vi "ADC INL_sweep.vi"(8 "error in (no error)":errorcluster, 9 "Sequence parameters":string[][](array[string])=[["Min limit", "Max limit", "Register sheet file", "Register Sheet"], ["", "", "CC2600.xls", "TX_BLE;Trim"], ["Reg write (addr;value)", "Operating frequency [Hz]", "", ""], ["NA", "2.44G", "", ""]], 10 "Run type":i32, 11 "Method parameters":T3={"Dev"={"Do not disturb DUT"=FALSE, "XOSC"=32000000.0, "Board type"="", "EM"="", "Configure tempboard"=TRUE, "Device specific info"=[], "Generic Object"=refnum}, "Method"={"Run type"=1, "Test name"="Current LPM2 4", "Comment"="", "Results folder"="", "AFC"=enum."Off", "Method name"="Current LPM2 4", "Method results"={"Excel brief report"=FALSE, "Spotfire report"=FALSE, "Starfish report"=FALSE}, "Operator"="", "Reference time"=timestamp(0 s since 1904-01-01), "AFC delay"=0.0, "Initialization"=enum."Enabled", "MD5 Sum"="", "HW addon board"=enum."None", "AFC Regsheet"="", "AFC Regfile"=path "", "dummy"=0.0}, "Inst"={"Instr"={"PS1"={"Name"="", "GPIB address"="", "VISA session"=""}, "PS2"={"Name"="", "GPIB address"="", "VISA session"=""}, "TC1"={"Name"="", "GPIB address"="", "VISA session"=""}, "TC2"={"Name"="", "GPIB address"="", "VISA session"=""}, "SA1"={"Name"="", "GPIB address"="", "VISA session"=""}, "SA2"={"Name"="", "GPIB address"="", "VISA session"=""}, "SG1"={"Name"="", "GPIB address"="", "VISA session"=""}, "SG2"={"Name"="", "GPIB address"="", "VISA session"=""}, "SG3"={"Name"="", "GPIB address"="", "VISA session"=""}, "MI1"={"Name"="", "GPIB address"="", "VISA session"=""}, "MI2"={"Name"="", "GPIB address"="", "VISA session"=""}, "SW SA"={"Name"="", "Controller addr"=""}, "SW SG"={"Name"="", "Controller addr"=""}, "MI3"={"Name"="", "GPIB address"="", "VISA session"=""}}, "Switchbox"={"RF Path"=0, "Cal compensation"=enum."TX", "Switchbox gain mode"="", "State"=enum."TX"}, "Instr to control (i.e. SA1)"="Default", "Intrument info string"=""}, "Sequence parameters"=[["Weight", "Min Limit", "Max Limit", "Register Sheet", "", "", "", "", "", "", "", "", ""], ["Vital", "", "1", "LPM2", "", "", "", "", "", "", "", "", ""], ["Resolution", "Reg write (addr;value)", "Chip mode", "Range", "", "", "", "", "", "", "", "", ""], ["u", "NA", "", "auto", "", "", "", "", "", "", "", "", ""]], "Cond"={"Temp logged"=25.0, "VDD1_PS1_6V"=-999.0, "VDD2_PS1_25V"=-999.0, "VDD4_PS2_25V"=-999.0, "VDD3_PS2_6V"=-999.0}, "Meas config"={"X-axis inner loop index"=32000000, "Y-axis outer loop index"=32000000, "X-axis"=[], "Y-axis"=[], "X-axis array req size"=32000000, "Y-axis array req size"=32000000, "Param description"=[], "Use meas clust for reporting"=FALSE, "Parameter index (page)"=0, "X-axis name"="", "Y-axis name"=""}} {"Cond"."VDD3_PS2_6V" format="%.3f"; "Cond"."VDD4_PS2_25V" format="%.3f"; "Cond"."VDD2_PS1_25V" format="%.3f"; "Cond"."VDD1_PS1_6V" format="%.3f"; "Method"."dummy" format="%.1p"; "Method"."AFC delay" format="%.1p"; "Dev"."XOSC" format="%.3p"}) -> (0 "error out":errorcluster, 1 "End method error":T2, 2 "Short Results":string[](array[string])=["0.00", "0.00", "0.00", "0.00"], 3 "Result summary":string[][](array[string])=[["Critical", "Output Power@2405 MHz", "-3", "4", "dBm"], ["Critical", "Output Power@2410 MHz", "-3", "4", "dBm"]])   [LabVIEW 2019]
doc: "[AutoDocStart]Performs crystal accuracy measurements. Measures the offset from ideal frequency. Primarily used for tuning XOSC capacitors and verifying XOSC trims.\n\nSweeping parameters: operating frequency, OSC override value and VDDR level\n\nResults: Offset frequency in ppm[AutoDocEnd]"
uses:
  User Lib/Utilities/Cluster definitions/DUT VDD1.ctl
  User Lib/Utilities/Cluster definitions/DUT VDD2.ctl
  User Lib/Utilities/Cluster definitions/DUT VDD3.ctl
  User Lib/Utilities/Cluster definitions/DUT VDD4.ctl
  User Lib/Utilities/Cluster definitions/DUT vdd control.ctl
  42f514b6-df04-40b6-a03b-a487344522a2.vi
  3f8b4189-43b3-45b7-8bba-bb7e10ae7045.vi
  47332434-656c-4693-9234-e05a15154894.vi
  62b45376-0a3e-4237-a030-b0a612edc8e5.vi
  b7ff9f93-cf4b-49d2-9220-d5c2ebaf56eb.vi
  9f9df643-cad2-47cb-a2d6-a9993951f146.vi
  0285ada5-cea9-4f7c-8e18-3c0901f4aec6.vi
  d5327cad-c336-4ca6-ac46-e2641e1e3ffd.vi
  User Lib/Utilities/Cluster definitions/Instr clust.ctl
  User Lib/Utilities/Cluster definitions/Method input.ctl
  User Lib/Utilities/Controls/Automatic Frequency Compensation types.ctl
  User Lib/Utilities/Controls/Method Reports.ctl
  User Lib/Utilities/Cluster definitions/End method error cluster.ctl
  User Lib/Utilities/Cluster definitions/Device specific info.ctl
  User Lib/Utilities/Cluster definitions/Method Initialization.ctl
  User Lib/Utilities/Switchbox control/SwitchBox_State._ENUMctl.ctl
  User Lib/Utilities/Controls/HW addon boards.ctl
panel:
  in  "Tab Control":T1(tab)
  # "°C"
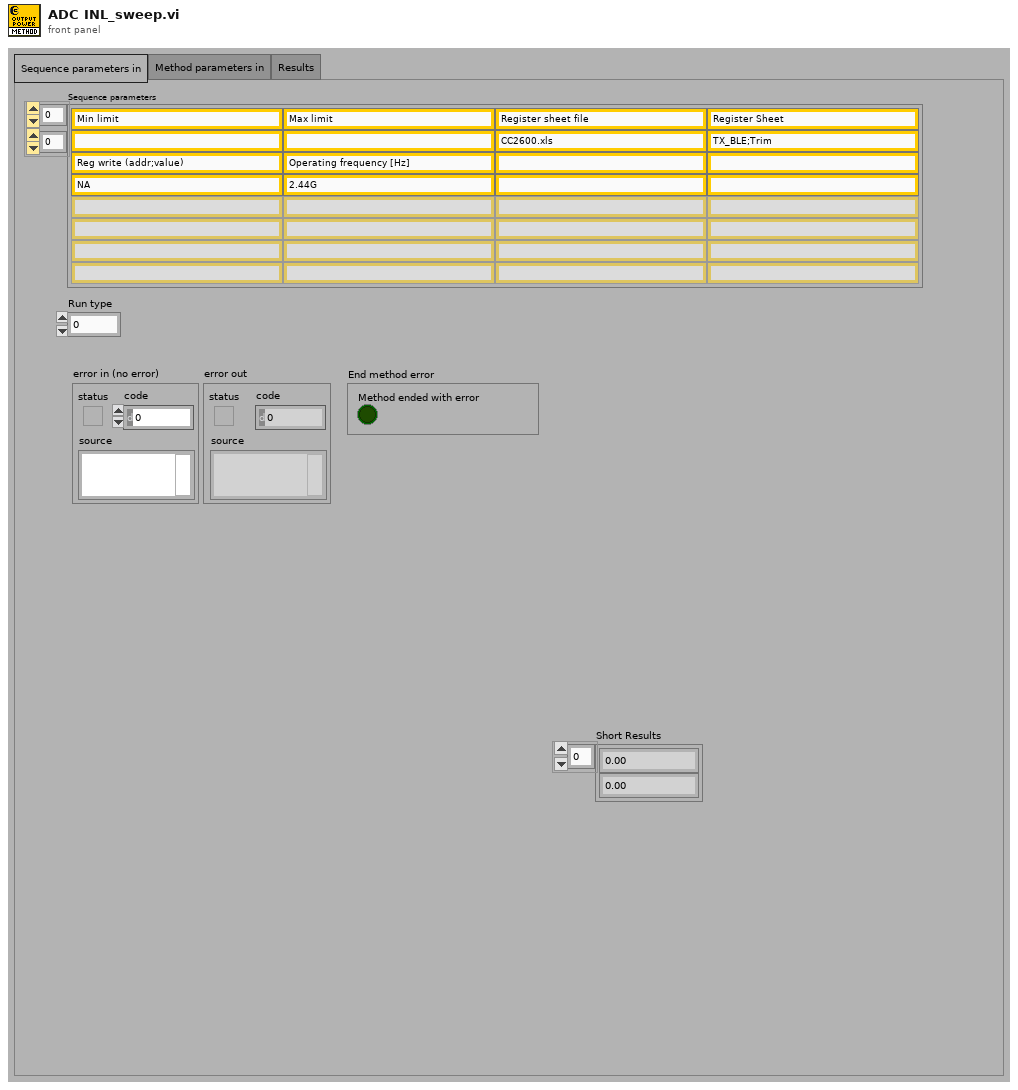
[diagram p1: front panel]
types:
  T1 = enum32{"Sequence parameters in", "Method parameters in", "Results"}
  T2 = typedef "End method error cluster.ctl" = cluster{"Method ended with error":bool}
  T3 = typedef "Method input.ctl" = cluster{"Dev":cluster{"Do not disturb DUT":bool, "XOSC":dbl, "Board type":string, "EM":string, "Configure tempboard":bool, "Device specific info":T4[], "Generic Object":refnum<class>}, "Method":cluster{"Run type":i32, "Test name":string, "Comment":string, "Results folder":string, "AFC":T5, "Method name":string, "Method results":T6, "Operator":string, "Reference time":timestamp, "AFC delay":dbl, "Initialization":T7, "MD5 Sum":string, "HW addon board":T8, "AFC Regsheet":string, "AFC Regfile":path, "dummy":dbl}, "Inst":T9, "Sequence parameters":string[][], "Cond":cluster{"Temp logged":dbl, "VDD1_PS1_6V":dbl, "VDD2_PS1_25V":dbl, "VDD4_PS2_25V":dbl, "VDD3_PS2_6V":dbl}, "Meas config":cluster{"X-axis inner loop index":i32, "Y-axis outer loop index":i32, "X-axis":string[], "Y-axis":string[], "X-axis array req size":i32, "Y-axis array req size":i32, "Param description":string[][], "Use meas clust for reporting":bool, "Parameter index (page)":i32, "X-axis name":string, "Y-axis name":string}}
  T4 = typedef "Device specific info.ctl" = cluster{"EM number":u8, "IP address":string, "Enabled":bool, "Slot no":u8, "RF path":u8, "EM name":string, "Wafer info":string, "AFC frequency ppm":dbl, "Register writes":string[][], "Meas data":string[][][], "Device comment":string}
  T5 = typedef "Automatic Frequency Compensation types.ctl" = enum16{"Off", "Compensate Instrument frequency", "Compensate DUT frequency", "Predictive - Compensate Instrument frequency", "Predictive - Compensate DUT frequency", "Do not skip re-init - Compensate Instrument frequency", "Do not skip re-init - Compensate DUT frequency"}
  T6 = typedef "Method Reports.ctl" = cluster{"Excel brief report":bool, "Spotfire report":bool, "Starfish report":bool}
  T7 = typedef "Method Initialization.ctl" = enum16{"Enabled", "Skip Instr and Device Init", "Enabled with Separate Flash", "Set PS, Device Init and Skip Instr Init", "Skip Device Init"}
  T8 = typedef "HW addon boards.ctl" = enum16{"None", "Current meas 5EM", "Stresstest 10EM"}
  T9 = typedef "Instr clust.ctl" = cluster{"Instr":cluster{"PS1":cluster{"Name":string, "GPIB address":string, "VISA session":refnum<visa-resource-name>}, "PS2":cluster{"Name":string, "GPIB address":string, "VISA session":refnum<visa-resource-name>}, "TC1":cluster{"Name":string, "GPIB address":string, "VISA session":refnum<visa-resource-name>}, "TC2":cluster{"Name":string, "GPIB address":string, "VISA session":refnum<visa-resource-name>}, "SA1":cluster{"Name":string, "GPIB address":string, "VISA session":refnum<visa-resource-name>}, "SA2":cluster{"Name":string, "GPIB address":string, "VISA session":refnum<visa-resource-name>}, "SG1":cluster{"Name":string, "GPIB address":string, "VISA session":refnum<visa-resource-name>}, "SG2":cluster{"Name":string, "GPIB address":string, "VISA session":refnum<visa-resource-name>}, "SG3":cluster{"Name":string, "GPIB address":string, "VISA session":refnum<visa-resource-name>}, "MI1":cluster{"Name":string, "GPIB address":string, "VISA session":refnum<visa-resource-name>}, "MI2":cluster{"Name":string, "GPIB address":string, "VISA session":refnum<visa-resource-name>}, "SW SA":cluster{"Name":string, "Controller addr":string}, "SW SG":cluster{"Name":string, "Controller addr":string}, "MI3":cluster{"Name":string, "GPIB address":string, "VISA session":refnum<visa-resource-name>}}, "Switchbox":cluster{"RF Path":i32, "Cal compensation":enum16{"TX", "RX", "Interferer", "No compensation", "Interferer2"}, "Switchbox gain mode":string, "State":T10}, "Instr to control (i.e. SA1)":string, "Intrument info string":string}
  T10 = typedef "SwitchBox_State._ENUMctl.ctl" = enum16{"TX", "RX", "SP:TX", "SP:RX", "SW:TX", "SW:RX"}
  T11 = typedef "DUT vdd control.ctl" = cluster{"VDD4 config":T12, "VDD3 config":T13, "VDD2 config":T14, "VDD1 config":T15}
  T12 = typedef "DUT VDD4.ctl" = u16
  T13 = typedef "DUT VDD3.ctl" = u16
  T14 = typedef "DUT VDD2.ctl" = u16
  T15 = typedef "DUT VDD1.ctl" = u16
  T16 = enum32{"NI Card Settings", "Memory Read Setting", "DC Capture", "ADC Ramp", "ADC Sine", "SNR", "Cap Calibration"}
  T17 = enum32{"Read from Memory", "Read .dat file", "NI Card Capture", "None"}
  T18 = cluster{"Path to Save plot":path, "Path to Raw Data plot":path}
  T19 = cluster{"Save INL/DNL Plot(Ramp)":bool, "Save SNR Plot":bool, "Save INL/DNL Plot(Sine)":bool, "Save INL/DNL Raw Data(Ramp)":bool, "Save SNR Raw Data":bool, "Save INL/DNL Raw Data(Sine)":bool, "Save DC Raw data":bool, "Save  Raw Data(Sine)":bool}
  T20 = cluster{"Min INL":dbl, "Max INL":dbl, "Min DNL":dbl, "Max DNL":dbl, "INL Range":dbl, "DNL Range":dbl, "Avg Hits/Code":dbl}
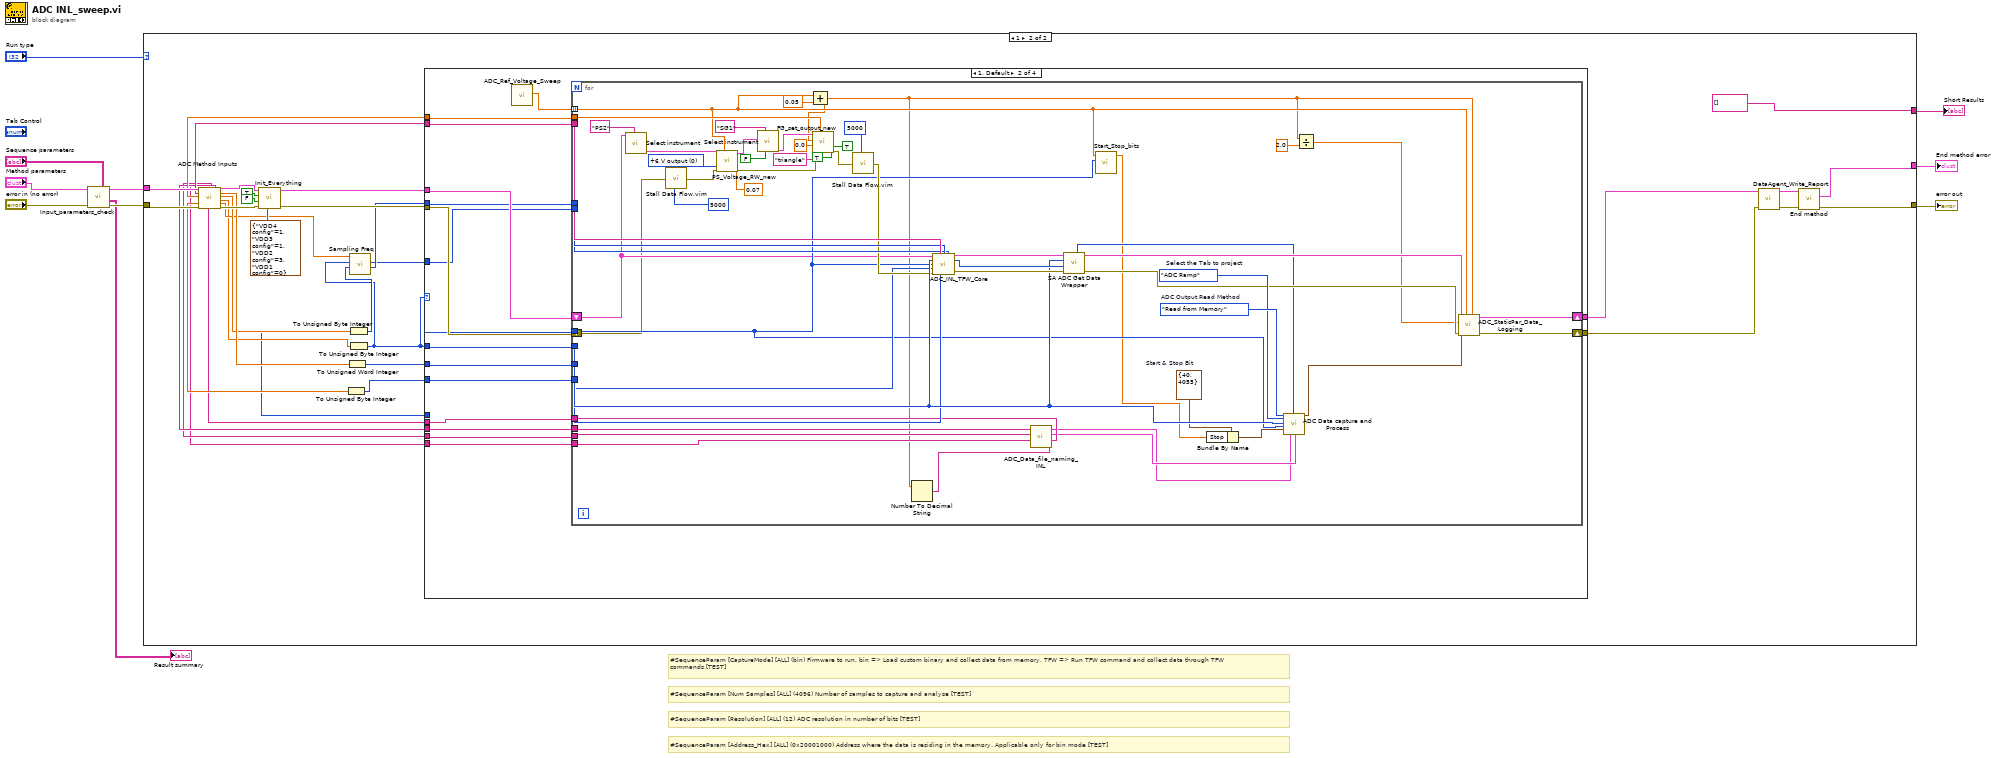
[diagram p0: block diagram]
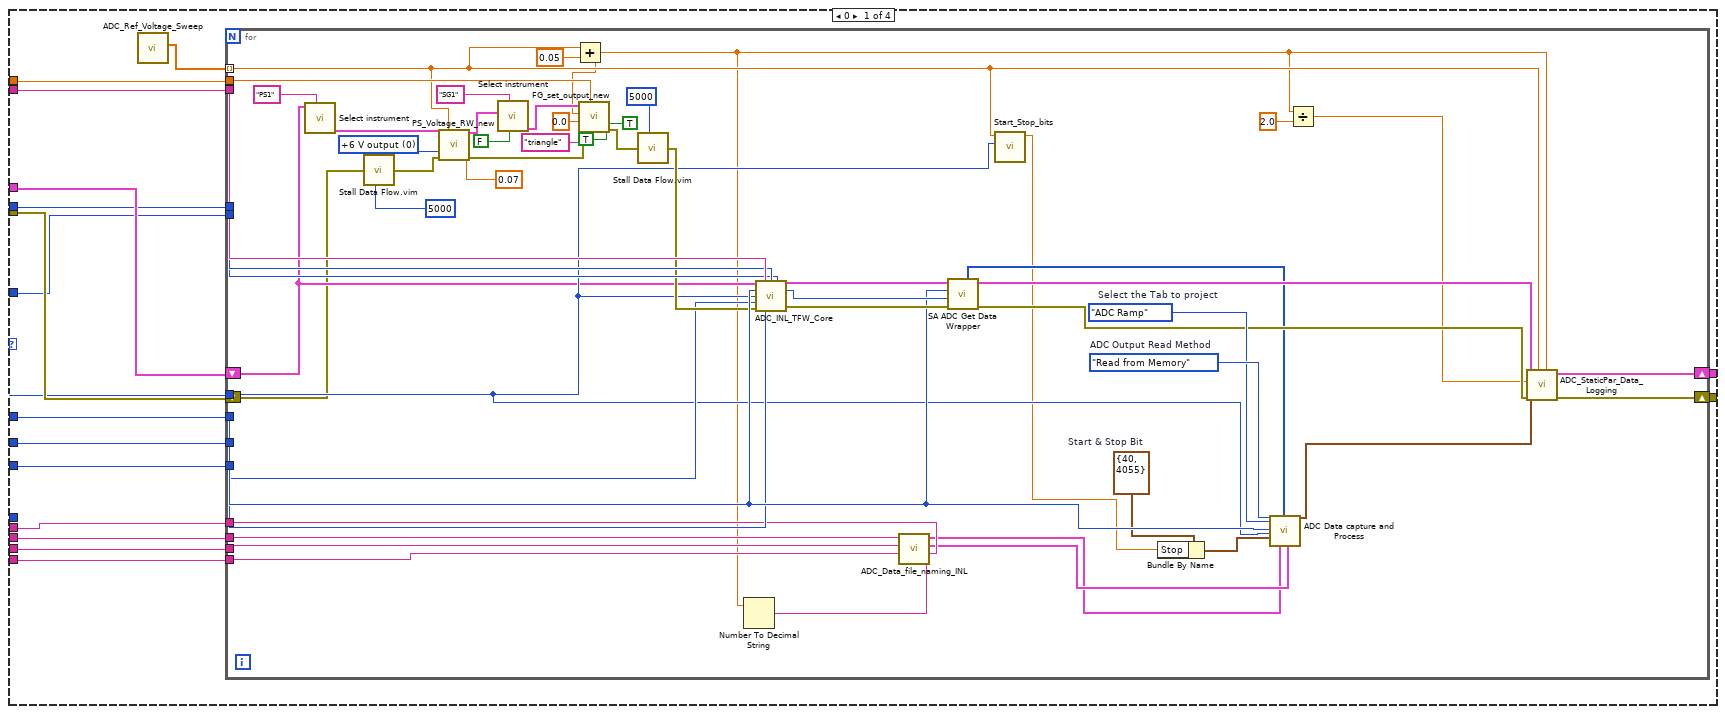
[diagram p3: hidden frame]
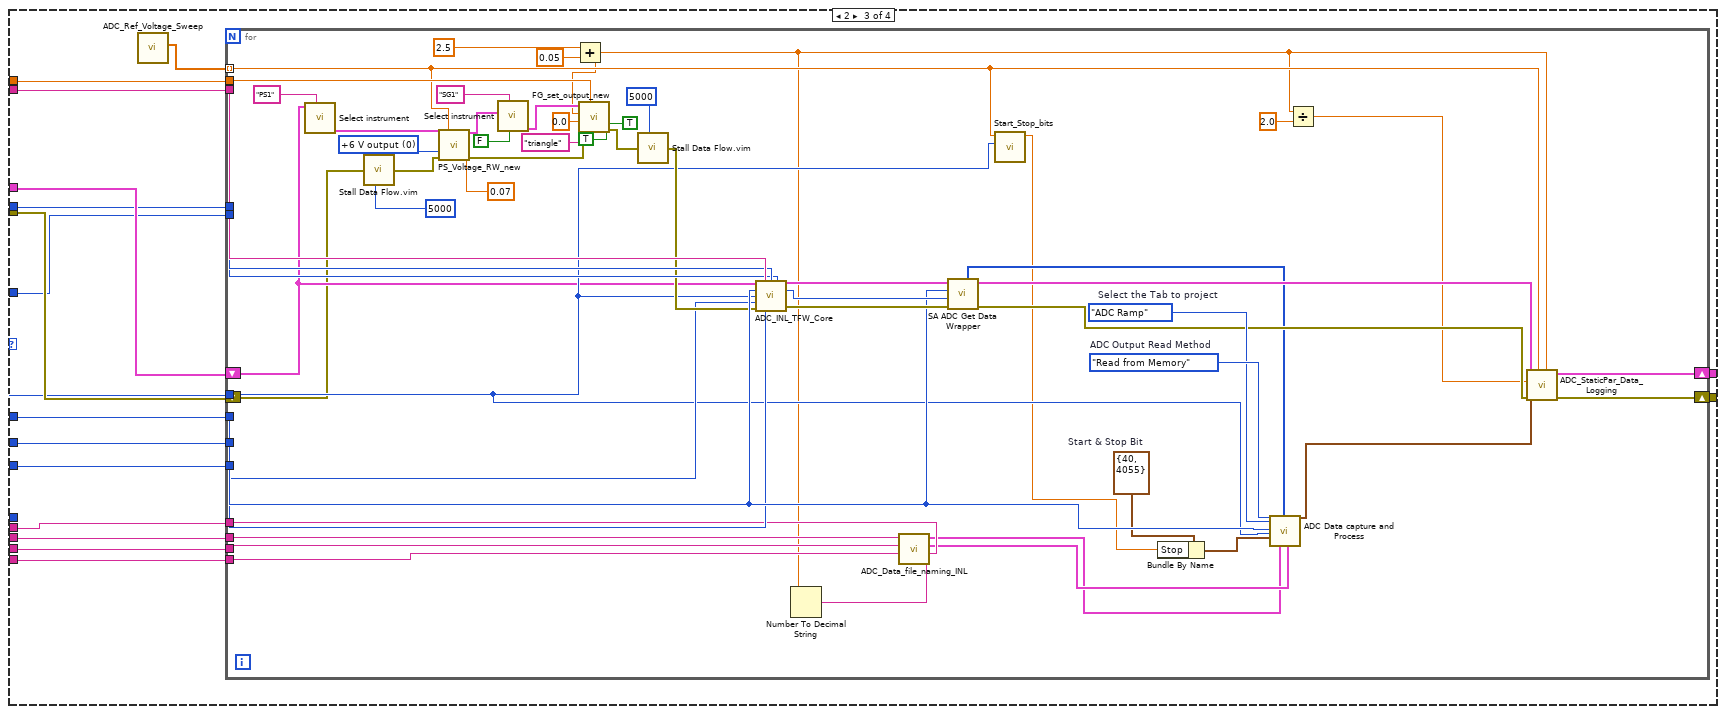
[diagram p4: hidden frame]
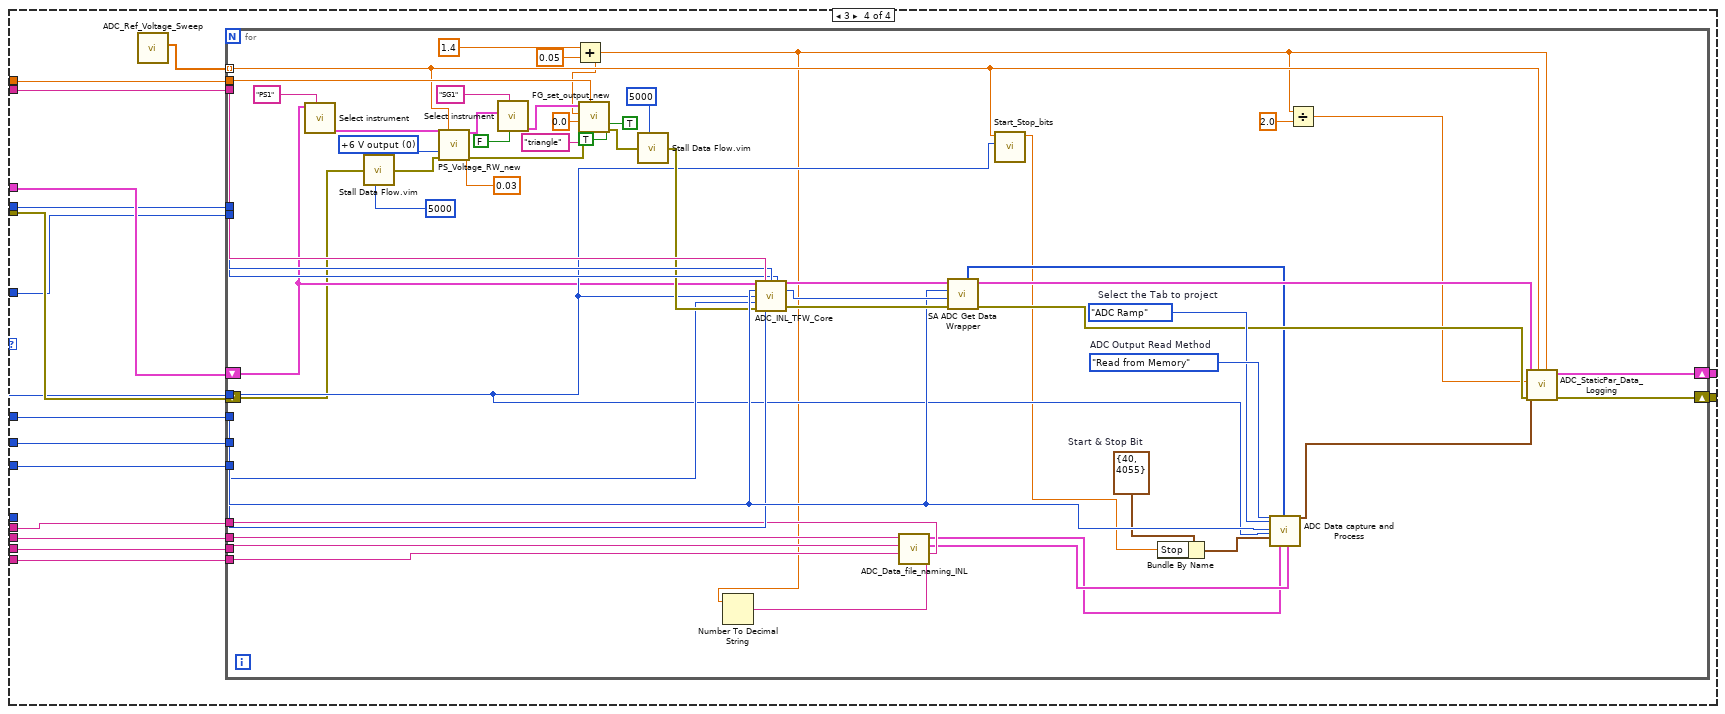
[diagram p5: hidden frame]
diagram:
  # "#SequenceParam [Num Samples] [ALL] (4096) Number of samples to capture and analyse [TEST]"
  # "#SequenceParam [CaptureMode] [ALL] (bin) Firmware to run. bin => Load custom binary and collect data from memory. TFW => Run TFW command and collect data through TFW commands [TEST]"
  # "#SequenceParam [Address_Hex] [ALL] (0x20001000) Address where the data is residing in the memory. Applicable only for bin mode [TEST]"
  # "#SequenceParam [Resolution] [ALL] (12) ADC resolution in number of bits [TEST]"
  n1 = call "Input_parameters_check.vi"("Sequence parameters"="Sequence parameters", "error in"="error in (no error)", "Method cluster in"="Method parameters") -> ("error out"=w9:errorcluster, "Result summary"=→"Result summary":string[][], "Method cluster out"=w5:T3)  [unwired: 6 in]
  n2 = case shown="1" "Run type" {
    tunnel: w9 -> [w11 w33]
    tunnel: [w11 w44] -> w10
    tunnel: w5 -> [_ w34]
    tunnel: [_ w43] -> w4
    tunnel: [_ string[] []] -> w1
    frame 0, Default {
      # "Run type 0 is only for formatting the result summary"
    }
    frame 1 {
      n3 = call "ADC Method Inputs.vi"("Method cluster in"=w34, "error in (no error)"=w33) -> ("Capture Mode"=w21:string, "Signal Freq"=w17:dbl, "ADC Chnl No."=w26:dbl, "Sampling Freq String"=w14:string, "Chnl No. string"=w13:string, "Resolution String"=w15:string, "Voltage Ref String"=w16:string, "Method cluster out"=w31:T3, "Num Samples"=w30:dbl, "Resolution"=w29:dbl, "Voltage Ref"=w27:dbl, "Sampling Freq"=w28:dbl, "error out"=w32:errorcluster)  [unwired: 3 in, 2 out]
      n4 = call "Init_Everything.vi"("VDD config"=T11 {"VDD4 config"=1, "VDD3 config"=1, "VDD2 config"=3, "VDD1 config"=0}, "error in"=w32, "Support current measurement?"=FALSE, "Override VDD Config"=TRUE, "Method cluster In"=w31) -> ("error out"=w25:errorcluster, "Method cluster out"=w12:T3)  [unwired: 3 in, 2 out]
      n5 = To Unsigned Byte Integer(number=w26) -> (unsigned 8bit integer=w22:u8)
      n6 = To Unsigned Word Integer(number=w30) -> (unsigned 16bit integer=w24:u16)
      n7 = To Unsigned Byte Integer(number=w29) -> (unsigned 8bit integer=w23:u8)
      n8 = To Unsigned Byte Integer(number=w27) -> (unsigned 8bit integer=w18:u8)
      n9 = call "Sampling Freq.vi"("Resolution"=w23, "Voltage Ref"=w18, "Sampling Freq"=w28) -> ("LGPT Count"=w20:u16, "SCOMP"=w19:u16)  [unwired: 7 in]
      n10 = case shown="1, Default" w18 {
        tunnel: [w61 w132 w203 w275] -> w38
        tunnel: [w60 w131 w202 w274] -> w37
        tunnel: w12 -> [w59 w130 w201 w273]
        tunnel: w25 -> [w58 w129 w200 w272]
        tunnel: w24 -> [w57 w128 w199 w271]
        tunnel: w23 -> [w56 w127 w198 w270]
        tunnel: w18 -> [w55 w126 w197 w269]
        tunnel: w22 -> [w54 w125 w196 w268]
        tunnel: w21 -> [w53 w124 w195 w267]
        tunnel: w20 -> [w52 w123 w194 w266]
        tunnel: w19 -> [w51 w122 w193 w265]
        tunnel: w17 -> [w49 w120 w191 w263]
        tunnel: w16 -> [w48 w119 w190 w262]
        tunnel: w15 -> [w47 w118 w189 w261]
        tunnel: w14 -> [w46 w117 w188 w260]
        tunnel: w13 -> [w45 w116 w187 w259]
        frame 0 {
          n11 = call "ADC_Ref_Voltage_Sweep.vi"() -> ("Ref voltage sweep"=w50:dbl[])  [unwired: 11 in]
          n12 = for {
            tunnel: w57 -> [w104]
            tunnel: w56 -> [w82]
            tunnel: w55 -> [w83]
            tunnel: w54 -> [w103]
            tunnel: w53 -> [w102]
            tunnel: w52 -> [w101]
            tunnel: w51 -> [w100]
            shift-right: [w110] -> w61
            shift-left: w59 -> [w76]
            shift-right: [w109] -> w60
            shift-left: w58 -> [w70]
            tunnel: w50 -> [w65] mode=indexing
            tunnel: w49 -> [w92]
            tunnel: w48 -> [w89]
            tunnel: w47 -> [w88]
            tunnel: w46 -> [w87]
            tunnel: w45 -> [w86]
            w77 = u16 0 items=["+6 V output", "+25 V output", "-25 V output", "ALL TERM"] ("Output Terminals")
            w81 = cluster{"Start":i32, "Stop":i32} {"Start"=40, "Stop"=4055}  # Start & Stop Bit
            w114 = T16."ADC Ramp"  # Select the Tab to project
            w115 = T17."Read from Memory"  # ADC Output Read Method
            n13 = call "Select instrument.vi"("Instr.Instr to control (i.e. SA1)"="PS1", "Method cluster in"=w76) -> ("Instr out"=w75:T9)  [unwired: 7 in, 2 out]
            n14 = call "Stall Data Flow.vim"("value in"=w70, "milliseconds to wait"=u32 5000) -> ("value out"=w71:errorcluster)  [unwired: 1 out]
            n15 = call "PS_Voltage_RW_new.vi"("InstrCluster in"=w75, "Set Voltage"=w65, "Current(0)"=0.07, "Output Terminals"=w77, "error in (no error)"=w71) -> ("InstrCluster out"=w74:T9, "error out"=w78:errorcluster)  [unwired: 8 in, 1 out]
            n16 = call "Select instrument.vi"("Method cluster (T) / Instr cluster (F)"=FALSE, "Instr.Instr to control (i.e. SA1)"="SG1", "Instr in"=w74) -> ("Instr out"=w99:T9)  [unwired: 6 in, 2 out]
            n17 = Add(x=w65, y=0.05) -> (x+y=w63:dbl)
            n18 = call "FG_set_output_new.vi"("High impedance (T)"=TRUE, "Enable Output?"=TRUE, "Function (DC, Sine, Square, Triangle, Ramp up, Ramp down, Pulse)"="triangle", "Frequency [Hz]"=w92, "error in"=w78, "Low voltage"=0.0, "High voltage (or DC)"=w63, "InstrCluster in"=w99) -> ("error out"=w97:errorcluster)  [unwired: 2 in, 1 out]
            n19 = call "Stall Data Flow.vim"("value in"=w97, "milliseconds to wait"=u32 5000) -> ("value out"=w96:errorcluster)  [unwired: 1 out]
            n20 = Number To Decimal String(number=w63) -> (decimal integer string=w64:string)  [unwired: 1 in]
            n21 = call "ADC_INL_TFW_Core.vi"("Method cluster in"=w76, "Capture Mode"=w102, "LGPT Count"=w101, "SCOMP"=w100, "No. Samples"=w104, "Resolution"=w82, "Voltage Ref"=w83, "error in"=w96, "ADC Chnl No."=w103) -> ("Method cluster out"=w106:T3, "ResPar[0] Data Address"=w105:u32, "error out"=w107:errorcluster)  [unwired: 3 in, 1 out]
            n22 = call "ADC_Data_file_naming_INL.vi"("Amplitude (Vpp)"=w64, "ADC Chn. No"=w86, "Sampling Freq String"=w87, "Resolution String"=w88, "Voltage Ref String"=w89) -> ("path to save"=w85:T18, "Save data"=w84:T19)  [unwired: 5 in]
            n23 = call "SA ADC Get Data Wrapper.vi"("error in"=w107, "Data Address"=w105, "Num Samples"=w104, "Method cluster in"=w106) -> ("error out"=w113:errorcluster, "output cluster"=w112:T3, "ADC samples"=w111:u32[])  [unwired: 2 in, 3 out]
            n24 = call "Start_Stop_bits.vi"("Resolution"=w82, "Input Amplitude"=w65) -> ("Stop Bit"=w79:dbl)  [unwired: 9 in]
            n25 = Bundle By Name(cluster=w81, "Stop"=w79) -> (w80:cluster{"Start":i32, "Stop":i32})
            n26 = call "ADC Data capture and Process.vi"("ADC Output Read Method"=w115, "Select the Tab to project"=w114, "No.of samples"=w104, "Resolution"=w82, "Start & Stop Bit"=w80, "Save data"=w84, "Input Waveform"=w111, "path to save"=w85) -> ("Static Parameters (Ramp)"=w108:T20)  [unwired: 14 in, 5 out]
            n27 = Divide(x=w63, y=2.0) -> (x/y=w67:dbl)
            n28 = call "ADC_StaticPar_Data_Logging.vi"("Offset (V)"=w67, "Amplitude (Vpp)"=w63, "Ref Voltage"=w65, "error in (no error)"=w113, "Static Parameters (Ramp)"=w108, "output cluster"=w112) -> ("error out"=w109:errorcluster, "Method cluster out"=w110:T3)  [unwired: 4 in]
          }
        }
        frame 1, Default {
          n29 = call "ADC_Ref_Voltage_Sweep.vi"() -> ("Ref voltage sweep"=w121:dbl[])  [unwired: 11 in]
          n30 = for {
            tunnel: w128 -> [w175]
            tunnel: w127 -> [w153]
            tunnel: w126 -> [w154]
            tunnel: w125 -> [w174]
            tunnel: w124 -> [w173]
            tunnel: w123 -> [w172]
            tunnel: w122 -> [w171]
            shift-right: [w181] -> w132
            shift-left: w130 -> [w147]
            shift-right: [w180] -> w131
            shift-left: w129 -> [w141]
            tunnel: w121 -> [w136] mode=indexing
            tunnel: w120 -> [w163]
            tunnel: w119 -> [w160]
            tunnel: w118 -> [w159]
            tunnel: w117 -> [w158]
            tunnel: w116 -> [w157]
            w148 = u16 0 items=["+6 V output", "+25 V output", "-25 V output", "ALL TERM"] ("Output Terminals")
            w152 = cluster{"Start":i32, "Stop":i32} {"Start"=40, "Stop"=4055}  # Start & Stop Bit
            w185 = T16."ADC Ramp"  # Select the Tab to project
            w186 = T17."Read from Memory"  # ADC Output Read Method
            n31 = call "Select instrument.vi"("Instr.Instr to control (i.e. SA1)"="PS2", "Method cluster in"=w147) -> ("Instr out"=w146:T9)  [unwired: 7 in, 2 out]
            n32 = call "Stall Data Flow.vim"("value in"=w141, "milliseconds to wait"=u32 5000) -> ("value out"=w142:errorcluster)  [unwired: 1 out]
            n33 = call "PS_Voltage_RW_new.vi"("InstrCluster in"=w146, "Set Voltage"=w136, "Current(0)"=0.07, "Output Terminals"=w148, "error in (no error)"=w142) -> ("InstrCluster out"=w145:T9, "error out"=w149:errorcluster)  [unwired: 8 in, 1 out]
            n34 = call "Select instrument.vi"("Method cluster (T) / Instr cluster (F)"=FALSE, "Instr.Instr to control (i.e. SA1)"="SG1", "Instr in"=w145) -> ("Instr out"=w170:T9)  [unwired: 6 in, 2 out]
            n35 = Add(x=w136, y=0.05) -> (x+y=w134:dbl)
            n36 = call "FG_set_output_new.vi"("High impedance (T)"=TRUE, "Enable Output?"=TRUE, "Function (DC, Sine, Square, Triangle, Ramp up, Ramp down, Pulse)"="triangle", "Frequency [Hz]"=w163, "error in"=w149, "Low voltage"=0.0, "High voltage (or DC)"=w134, "InstrCluster in"=w170) -> ("error out"=w168:errorcluster)  [unwired: 2 in, 1 out]
            n37 = call "Stall Data Flow.vim"("value in"=w168, "milliseconds to wait"=u32 5000) -> ("value out"=w167:errorcluster)  [unwired: 1 out]
            n38 = Number To Decimal String(number=w134) -> (decimal integer string=w135:string)  [unwired: 1 in]
            n39 = call "ADC_INL_TFW_Core.vi"("Method cluster in"=w147, "Capture Mode"=w173, "LGPT Count"=w172, "SCOMP"=w171, "No. Samples"=w175, "Resolution"=w153, "Voltage Ref"=w154, "error in"=w167, "ADC Chnl No."=w174) -> ("Method cluster out"=w177:T3, "ResPar[0] Data Address"=w176:u32, "error out"=w178:errorcluster)  [unwired: 3 in, 1 out]
            n40 = call "ADC_Data_file_naming_INL.vi"("Amplitude (Vpp)"=w135, "ADC Chn. No"=w157, "Sampling Freq String"=w158, "Resolution String"=w159, "Voltage Ref String"=w160) -> ("path to save"=w156:T18, "Save data"=w155:T19)  [unwired: 5 in]
            n41 = call "SA ADC Get Data Wrapper.vi"("error in"=w178, "Data Address"=w176, "Num Samples"=w175, "Method cluster in"=w177) -> ("error out"=w184:errorcluster, "output cluster"=w183:T3, "ADC samples"=w182:u32[])  [unwired: 2 in, 3 out]
            n42 = call "Start_Stop_bits.vi"("Resolution"=w153, "Input Amplitude"=w136) -> ("Stop Bit"=w150:dbl)  [unwired: 9 in]
            n43 = Bundle By Name(cluster=w152, "Stop"=w150) -> (w151:cluster{"Start":i32, "Stop":i32})
            n44 = call "ADC Data capture and Process.vi"("ADC Output Read Method"=w186, "Select the Tab to project"=w185, "No.of samples"=w175, "Resolution"=w153, "Start & Stop Bit"=w151, "Save data"=w155, "Input Waveform"=w182, "path to save"=w156) -> ("Static Parameters (Ramp)"=w179:T20)  [unwired: 14 in, 5 out]
            n45 = Divide(x=w134, y=2.0) -> (x/y=w138:dbl)
            n46 = call "ADC_StaticPar_Data_Logging.vi"("Offset (V)"=w138, "Amplitude (Vpp)"=w134, "Ref Voltage"=w136, "error in (no error)"=w184, "Static Parameters (Ramp)"=w179, "output cluster"=w183) -> ("error out"=w180:errorcluster, "Method cluster out"=w181:T3)  [unwired: 4 in]
          }
        }
        frame 2 {
          n47 = call "ADC_Ref_Voltage_Sweep.vi"() -> ("Ref voltage sweep"=w192:dbl[])  [unwired: 11 in]
          n48 = for {
            tunnel: w199 -> [w247]
            tunnel: w198 -> [w225]
            tunnel: w197 -> [w226]
            tunnel: w196 -> [w246]
            tunnel: w195 -> [w245]
            tunnel: w194 -> [w244]
            tunnel: w193 -> [w243]
            shift-right: [w253] -> w203
            shift-left: w201 -> [w219]
            shift-right: [w252] -> w202
            shift-left: w200 -> [w213]
            tunnel: w192 -> [w208] mode=indexing
            tunnel: w191 -> [w235]
            tunnel: w190 -> [w232]
            tunnel: w189 -> [w231]
            tunnel: w188 -> [w230]
            tunnel: w187 -> [w229]
            w220 = u16 0 items=["+6 V output", "+25 V output", "-25 V output", "ALL TERM"] ("Output Terminals")
            w224 = cluster{"Start":i32, "Stop":i32} {"Start"=40, "Stop"=4055}  # Start & Stop Bit
            w257 = T16."ADC Ramp"  # Select the Tab to project
            w258 = T17."Read from Memory"  # ADC Output Read Method
            n49 = call "Select instrument.vi"("Instr.Instr to control (i.e. SA1)"="PS1", "Method cluster in"=w219) -> ("Instr out"=w218:T9)  [unwired: 7 in, 2 out]
            n50 = call "Stall Data Flow.vim"("value in"=w213, "milliseconds to wait"=u32 5000) -> ("value out"=w214:errorcluster)  [unwired: 1 out]
            n51 = call "PS_Voltage_RW_new.vi"("InstrCluster in"=w218, "Set Voltage"=w208, "Current(0)"=0.07, "Output Terminals"=w220, "error in (no error)"=w214) -> ("InstrCluster out"=w217:T9, "error out"=w221:errorcluster)  [unwired: 8 in, 1 out]
            n52 = call "Select instrument.vi"("Method cluster (T) / Instr cluster (F)"=FALSE, "Instr.Instr to control (i.e. SA1)"="SG1", "Instr in"=w217) -> ("Instr out"=w242:T9)  [unwired: 6 in, 2 out]
            n53 = Add(x=2.5, y=0.05) -> (x+y=w205:dbl)
            n54 = call "FG_set_output_new.vi"("High impedance (T)"=TRUE, "Enable Output?"=TRUE, "Function (DC, Sine, Square, Triangle, Ramp up, Ramp down, Pulse)"="triangle", "Frequency [Hz]"=w235, "error in"=w221, "Low voltage"=0.0, "High voltage (or DC)"=w205, "InstrCluster in"=w242) -> ("error out"=w240:errorcluster)  [unwired: 2 in, 1 out]
            n55 = call "Stall Data Flow.vim"("value in"=w240, "milliseconds to wait"=u32 5000) -> ("value out"=w239:errorcluster)  [unwired: 1 out]
            n56 = call "ADC_INL_TFW_Core.vi"("Method cluster in"=w219, "Capture Mode"=w245, "LGPT Count"=w244, "SCOMP"=w243, "No. Samples"=w247, "Resolution"=w225, "Voltage Ref"=w226, "error in"=w239, "ADC Chnl No."=w246) -> ("Method cluster out"=w249:T3, "ResPar[0] Data Address"=w248:u32, "error out"=w250:errorcluster)  [unwired: 3 in, 1 out]
            n57 = Number To Decimal String(number=w205) -> (decimal integer string=w206:string)  [unwired: 1 in]
            n58 = call "ADC_Data_file_naming_INL.vi"("Amplitude (Vpp)"=w206, "ADC Chn. No"=w229, "Sampling Freq String"=w230, "Resolution String"=w231, "Voltage Ref String"=w232) -> ("path to save"=w228:T18, "Save data"=w227:T19)  [unwired: 5 in]
            n59 = call "SA ADC Get Data Wrapper.vi"("error in"=w250, "Data Address"=w248, "Num Samples"=w247, "Method cluster in"=w249) -> ("error out"=w256:errorcluster, "output cluster"=w255:T3, "ADC samples"=w254:u32[])  [unwired: 2 in, 3 out]
            n60 = call "Start_Stop_bits.vi"("Resolution"=w225, "Input Amplitude"=w208) -> ("Stop Bit"=w222:dbl)  [unwired: 9 in]
            n61 = Bundle By Name(cluster=w224, "Stop"=w222) -> (w223:cluster{"Start":i32, "Stop":i32})
            n62 = call "ADC Data capture and Process.vi"("ADC Output Read Method"=w258, "Select the Tab to project"=w257, "No.of samples"=w247, "Resolution"=w225, "Start & Stop Bit"=w223, "Save data"=w227, "Input Waveform"=w254, "path to save"=w228) -> ("Static Parameters (Ramp)"=w251:T20)  [unwired: 14 in, 5 out]
            n63 = Divide(x=w205, y=2.0) -> (x/y=w210:dbl)
            n64 = call "ADC_StaticPar_Data_Logging.vi"("Offset (V)"=w210, "Amplitude (Vpp)"=w205, "Ref Voltage"=w208, "error in (no error)"=w256, "Static Parameters (Ramp)"=w251, "output cluster"=w255) -> ("error out"=w252:errorcluster, "Method cluster out"=w253:T3)  [unwired: 4 in]
          }
        }
        frame 3 {
          n65 = call "ADC_Ref_Voltage_Sweep.vi"() -> ("Ref voltage sweep"=w264:dbl[])  [unwired: 11 in]
          n66 = for {
            tunnel: w271 -> [w319]
            tunnel: w270 -> [w297]
            tunnel: w269 -> [w298]
            tunnel: w268 -> [w318]
            tunnel: w267 -> [w317]
            tunnel: w266 -> [w316]
            tunnel: w265 -> [w315]
            shift-right: [w325] -> w275
            shift-left: w273 -> [w291]
            shift-right: [w324] -> w274
            shift-left: w272 -> [w285]
            tunnel: w264 -> [w280] mode=indexing
            tunnel: w263 -> [w307]
            tunnel: w262 -> [w304]
            tunnel: w261 -> [w303]
            tunnel: w260 -> [w302]
            tunnel: w259 -> [w301]
            w292 = u16 0 items=["+6 V output", "+25 V output", "-25 V output", "ALL TERM"] ("Output Terminals")
            w296 = cluster{"Start":i32, "Stop":i32} {"Start"=40, "Stop"=4055}  # Start & Stop Bit
            w329 = T16."ADC Ramp"  # Select the Tab to project
            w330 = T17."Read from Memory"  # ADC Output Read Method
            n67 = call "Select instrument.vi"("Instr.Instr to control (i.e. SA1)"="PS1", "Method cluster in"=w291) -> ("Instr out"=w290:T9)  [unwired: 7 in, 2 out]
            n68 = call "Stall Data Flow.vim"("value in"=w285, "milliseconds to wait"=u32 5000) -> ("value out"=w286:errorcluster)  [unwired: 1 out]
            n69 = call "PS_Voltage_RW_new.vi"("InstrCluster in"=w290, "Set Voltage"=w280, "Current(0)"=0.03, "Output Terminals"=w292, "error in (no error)"=w286) -> ("InstrCluster out"=w289:T9, "error out"=w293:errorcluster)  [unwired: 8 in, 1 out]
            n70 = call "Select instrument.vi"("Method cluster (T) / Instr cluster (F)"=FALSE, "Instr.Instr to control (i.e. SA1)"="SG1", "Instr in"=w289) -> ("Instr out"=w314:T9)  [unwired: 6 in, 2 out]
            n71 = Add(x=1.4, y=0.05) -> (x+y=w277:dbl)
            n72 = call "FG_set_output_new.vi"("High impedance (T)"=TRUE, "Enable Output?"=TRUE, "Function (DC, Sine, Square, Triangle, Ramp up, Ramp down, Pulse)"="triangle", "Frequency [Hz]"=w307, "error in"=w293, "Low voltage"=0.0, "High voltage (or DC)"=w277, "InstrCluster in"=w314) -> ("error out"=w312:errorcluster)  [unwired: 2 in, 1 out]
            n73 = call "Stall Data Flow.vim"("value in"=w312, "milliseconds to wait"=u32 5000) -> ("value out"=w311:errorcluster)  [unwired: 1 out]
            n74 = Number To Decimal String(number=w277) -> (decimal integer string=w278:string)  [unwired: 1 in]
            n75 = call "ADC_INL_TFW_Core.vi"("Method cluster in"=w291, "Capture Mode"=w317, "LGPT Count"=w316, "SCOMP"=w315, "No. Samples"=w319, "Resolution"=w297, "Voltage Ref"=w298, "error in"=w311, "ADC Chnl No."=w318) -> ("Method cluster out"=w321:T3, "ResPar[0] Data Address"=w320:u32, "error out"=w322:errorcluster)  [unwired: 3 in, 1 out]
            n76 = call "ADC_Data_file_naming_INL.vi"("Amplitude (Vpp)"=w278, "ADC Chn. No"=w301, "Sampling Freq String"=w302, "Resolution String"=w303, "Voltage Ref String"=w304) -> ("path to save"=w300:T18, "Save data"=w299:T19)  [unwired: 5 in]
            n77 = call "SA ADC Get Data Wrapper.vi"("error in"=w322, "Data Address"=w320, "Num Samples"=w319, "Method cluster in"=w321) -> ("error out"=w328:errorcluster, "output cluster"=w327:T3, "ADC samples"=w326:u32[])  [unwired: 2 in, 3 out]
            n78 = call "Start_Stop_bits.vi"("Resolution"=w297, "Input Amplitude"=w280) -> ("Stop Bit"=w294:dbl)  [unwired: 9 in]
            n79 = Bundle By Name(cluster=w296, "Stop"=w294) -> (w295:cluster{"Start":i32, "Stop":i32})
            n80 = call "ADC Data capture and Process.vi"("ADC Output Read Method"=w330, "Select the Tab to project"=w329, "No.of samples"=w319, "Resolution"=w297, "Start & Stop Bit"=w295, "Save data"=w299, "Input Waveform"=w326, "path to save"=w300) -> ("Static Parameters (Ramp)"=w323:T20)  [unwired: 14 in, 5 out]
            n81 = Divide(x=w277, y=2.0) -> (x/y=w282:dbl)
            n82 = call "ADC_StaticPar_Data_Logging.vi"("Offset (V)"=w282, "Amplitude (Vpp)"=w277, "Ref Voltage"=w280, "error in (no error)"=w328, "Static Parameters (Ramp)"=w323, "output cluster"=w327) -> ("error out"=w324:errorcluster, "Method cluster out"=w325:T3)  [unwired: 4 in]
          }
        }
      }
      n83 = call "DataAgent_Write_Report.vi"("error in (no error)"=w37, "Method cluster in"=w38) -> ("error out"=w41:errorcluster, "Method cluster out"=w40:T3)  [unwired: 8 in]
      n84 = call "End method.vi"("error in"=w41, "Method cluster in"=w40) -> ("error out"=w44:errorcluster, "End method error"=w43:T2)  [unwired: 7 in, 1 out]
    }
  }
  "error out" <- w10
  "End method error" <- w4
  "Short Results" <- w1
